vi "OAT Polar PG Autoscale Polar as Needed.vi"(1 "polar attributes":T1={"maximum"=1.0, "minimum"=0.0, "clip to min"=FALSE, "log"=FALSE, "grid color"=0, "plot color"=0, "fmt and prec"={"format"=enum."Decimal", "precision"=2}, "visible section"=8} {"minimum" format="%.2f"; "maximum" format="%.2f"}, 2 "data":cluster{"magnitude":dbl, "phase":dbl}[](array[cluster]) {"phase" format="%.2f"; "magnitude" format="%.2f"}) -> (0 "polar attributes":T1={"maximum"=1.0, "minimum"=0.0, "clip to min"=FALSE, "log"=FALSE, "grid color"=0, "plot color"=0, "fmt and prec"={"format"=enum."Decimal", "precision"=2}, "visible section"=8} {"minimum" format="%.2f"; "maximum" format="%.2f"})   [LabVIEW 2017]
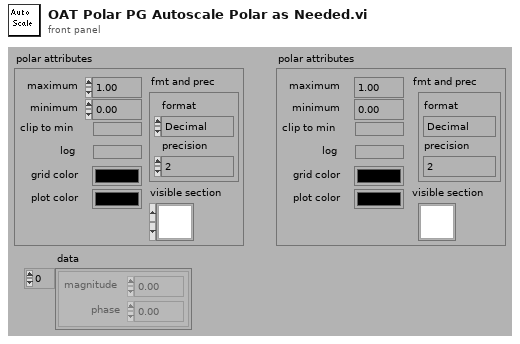
[diagram p1: front panel]
types:
  T1 = cluster{"maximum":dbl, "minimum":dbl, "clip to min":bool, "log":bool, "grid color":u32, "plot color":u32, "fmt and prec":cluster{"format":enum8{"Decimal", "Scientific", "Engineering", "Binary", "Octal", "Hex"}, "precision":u8}, "visible section":u16}
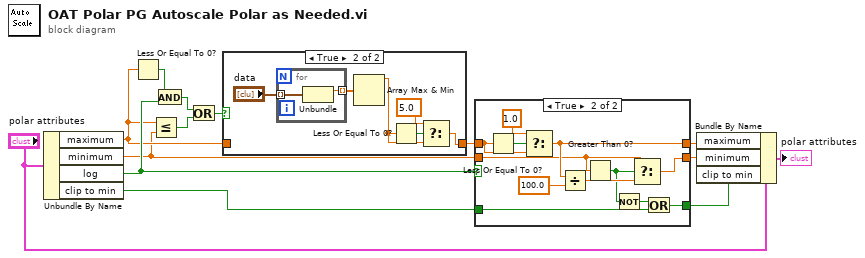
[diagram p0: block diagram]
diagram:
  n1 = Unbundle By Name("polar attributes") -> ("maximum"=w5:dbl, "minimum"=w4:dbl, "log"=w7:bool, "clip to min"=w1:bool)
  n2 = Less Or Equal To 0?(x=w5) -> (x <= 0?=w6:bool)
  n3 = Less Or Equal?(x=w5, y=w4) -> (x <= y?=w9:bool)
  n4 = And(x=w6, y=w7) -> (x .and. y?=w10:bool)
  n5 = Or(x=w10, y=w9) -> (x .or. y?=w8:bool)
  n6 = case shown="True" w8 {
    tunnel: w5 -> [w15 _]
    tunnel: [w15 w18] -> w11
    frame False {
    }
    frame True {
      n7 = for {
        tunnel: "data" -> [w23] mode=indexing
        tunnel: [w22] -> w21 mode=indexing
        n8 = Unbundle(w23) -> ("magnitude"=w22:dbl)  [unwired: 1 out]
      }
      n9 = Array Max & Min(array=w21) -> (max value=w16:dbl)  [unwired: 3 out]
      n10 = Less Or Equal To 0?(x=w16) -> (x <= 0?=w19:bool)
      n11 = Select(t=5.0, s=w19, f=w16) -> (s? t:f=w18:dbl)
    }
  }
  n12 = case shown="True" w7 {
    tunnel: w4 -> [w26 w33]
    tunnel: [w26 w32] -> w12
    tunnel: w11 -> [w25 w36]
    tunnel: [w25 w34] -> w3
    tunnel: [w24 w28] -> w2
    tunnel: w1 -> [w24 w29]
    frame False {
    }
    frame True {
      n13 = Less Or Equal To 0?(x=w36) -> (x <= 0?=w37:bool)
      n14 = Select(t=1.0, s=w37, f=w36) -> (s? t:f=w34:dbl)
      n15 = Divide(x=w34, y=100.0) -> (x/y=w31:dbl)
      n16 = Greater Than 0?(x=w33) -> (x > 0?=w30:bool)
      n17 = Not(x=w30) -> (.not. x?=w27:bool)
      n18 = Select(t=w33, s=w30, f=w31) -> (s? t:f=w32:dbl)
      n19 = Or(x=w27, y=w29) -> (x .or. y?=w28:bool)
    }
  }
  n20 = Bundle By Name(cluster="polar attributes", "maximum"=w3, "minimum"=w12, "clip to min"=w2) -> (→"polar attributes":T1)
